vi "SQLite File Path.vi"(8 "error in (no error)":errorcluster, 10 "SQLiteFileName":T1="Parameters.db", 11 "SQLite in":refnum<class "SQLite.lvclass">) -> (0 "error out":errorcluster, 2 "string":string, 3 "SQLite out":refnum<class "SQLite.lvclass">)   [LabVIEW 2021, in "SQLite.lvclass"]
uses:
  SQLite.lvclass
  SQLiteFileName.ctl
  SQLite.lvclass/SQLite.ctl
  vi.lib_New/TopPath/TopPath.lvlib
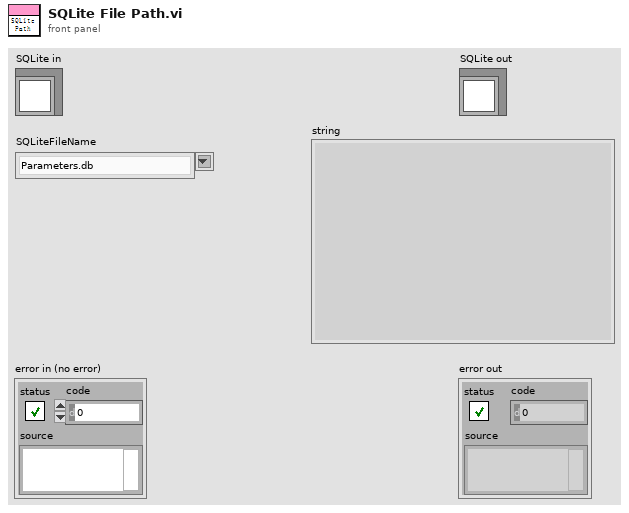
[diagram p1: front panel]
types:
  T1 = typedef "SQLite.lvclass/SQLiteFileName.ctl" = string
  T2 = typedef "TopPath.lvlib/Top Path.ctl" = cluster{"LV Source":path, "FilePath":path, "Data":path}
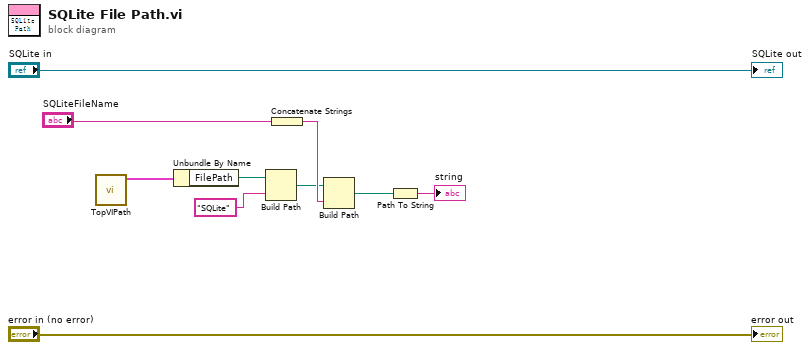
[diagram p0: block diagram]
diagram:
  n1 = call "TopVIPath.vi"() -> ("TopPath"=w1:T2)  [unwired: 10 in, 1 out]
  n2 = Unbundle By Name(w1) -> ("FilePath"=w7:path)
  n3 = Build Path(base path=w7, name or relative path="SQLite") -> (appended path=w6:path)
  n4 = Concatenate Strings("SQLiteFileName") -> (w8:string)
  n5 = Build Path(base path=w6, name or relative path=w8) -> (appended path=w4:path)
  n6 = Path To String(path=w4) -> (string=→"string":string)
  "error out" <- "error in (no error)"
  "SQLite out" <- "SQLite in"
